vi "Slide.vi"(8 "Center of Mass X2":dbl, 9 "Center of Mass X1":dbl) -> (2 "1, 0, -1":i32, 3 "Center of Mass avg.":dbl)   [LabVIEW 2014]
doc: "-1 - Left\n0 - Do Nothing\n1 - Right"
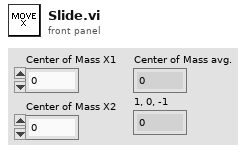
[diagram p1: front panel]
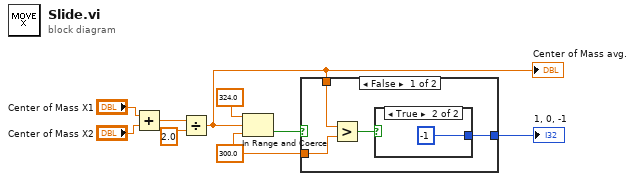
[diagram p0: block diagram]
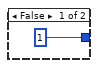
[diagram p2: hidden frame]
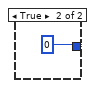
[diagram p3: hidden frame]
diagram:
  w2 = 300.0 ("lower limit")
  n1 = Add(x="Center of Mass X1", y="Center of Mass X2") -> (x+y=w7:dbl)
  n2 = Divide(x=w7, y=2.0) -> (x/y=w3:dbl)
  "Center of Mass avg." <- w3
  n3 = In Range and Coerce(upper limit=324.0, x=w3, lower limit=w2) -> (In Range?=w4:bool)  [unwired: 1 out]
  n4 = case shown="False" w4 {
    tunnel: w3 -> [w13 _]
    tunnel: w2 -> [w12 _]
    tunnel: [w10 0] -> w1
    frame False {
      n5 = Greater?(x=w13, y=w12) -> (0:w11:bool)
      n6 = case shown="True" w11 {
        tunnel: [1 -1] -> w10
        frame False {
        }
        frame True {
        }
      }
    }
    frame True {
    }
  }
  "1, 0, -1" <- w1
